vi "Collect.vi"(8 "error in (no error)":errorcluster, 11 "Disk Collector in":refnum<class "Disk Collector.lvclass">) -> (0 "error out":errorcluster, 2 "Metrics":refnum<data-value>[](array[refnum]), 3 "Disk Collector out":refnum<class "Disk Collector.lvclass">)   [LabVIEW 2020, in "Disk Collector.lvclass"]
uses:
  Disk Collector.lvclass
  C:/Github-locals/PromVIEW/src/collector/generic collector/Default Collector.lvclass
  src/metrics/metric/Metric.lvclass
  src/metrics/gauge/Gauge.lvclass
  Disk Collector.lvclass/Disk Collector.ctl
  src/collector/generic collector/Default Collector.lvclass
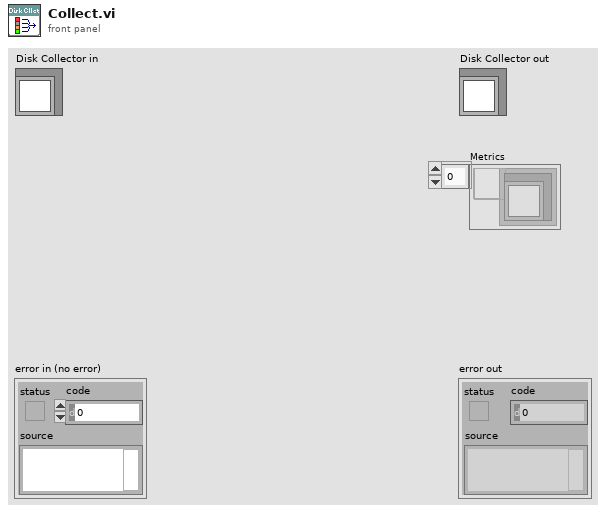
[diagram p1: front panel]
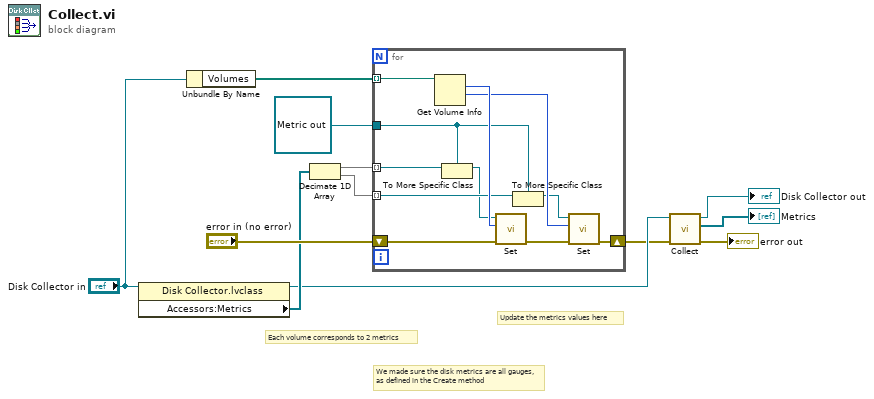
[diagram p0: block diagram]
diagram:
  # "Update the metrics values here"
  # "We made sure the disk metrics are all gauges, as defined in the Create method"
  # "Each volume corresponds to 2 metrics"
  n1 = property class="Disk Collector.lvclass"(reference="Disk Collector in") -> (reference out=w3:refnum<class "Disk Collector.lvclass">, "Accessors:Metrics"=w5:refnum<data-value>[])  [unwired: 1 in, 1 out]
  n2 = Unbundle By Name("Disk Collector in") -> ("Volumes"=w10:path[])
  n3 = Decimate 1D Array(w5) -> (w9:refnum<data-value>[], w8:refnum<data-value>[])
  n4 = for {
    tunnel: w10 -> [w23] mode=indexing
    tunnel: w9 -> [w17] mode=indexing
    tunnel: w8 -> [w16] mode=indexing
    shift-right: [w18] -> w1
    shift-left: "error in (no error)" -> [w19]
    tunnel: refnum<data-value> refnum ("Gauge Ref") -> [w15]
    n5 = Get Volume Info(11:w23) -> (1:w21:i64, 2:w22:i64)  [unwired: 1 in, 4 out]
    n6 = To More Specific Class(target class=w15, reference=w17) -> (specific class reference=w14:refnum<data-value>)  [unwired: 1 in, 1 out]
    n7 = call "Set.vi"("error in (no error)"=w19, "Value"=w22, "Gauge Ref"=w14) -> ("error out"=w20:errorcluster)  [unwired: 7 in, 1 out]
    n8 = To More Specific Class(target class=w15, reference=w16) -> (specific class reference=w13:refnum<data-value>)  [unwired: 1 in, 1 out]
    n9 = call "Set.vi"("error in (no error)"=w20, "Value"=w21, "Gauge Ref"=w13) -> ("error out"=w18:errorcluster)  [unwired: 7 in, 1 out]
  }
  n10 = call-parent "Collect.vi"("error in (no error)"=w1, "Default Collector in"=w3) -> ("error out"=→"error out":errorcluster, "Metrics"=→"Metrics":refnum<data-value>[], "Default Collector out"=→"Disk Collector out":refnum<class "Disk Collector.lvclass">)  [unwired: 7 in]
